vi "Configuration.vi"() -> ()   [LabVIEW 2018]
panel:
  out "error out":errorcluster
  in  "error in (no error)":errorcluster
  in  "Save":bool
  in  "Chromator COM":refnum<visa-resource-name>
  in  "Stop":bool
  in  "Merlin COM":refnum<visa-resource-name>
  in  "Source Meter COM":refnum<visa-resource-name>
  in  "Kaithely_PS COM":refnum<visa-resource-name>
  in  "Filter COM":refnum<visa-resource-name>
  # "Instrument Configuration"
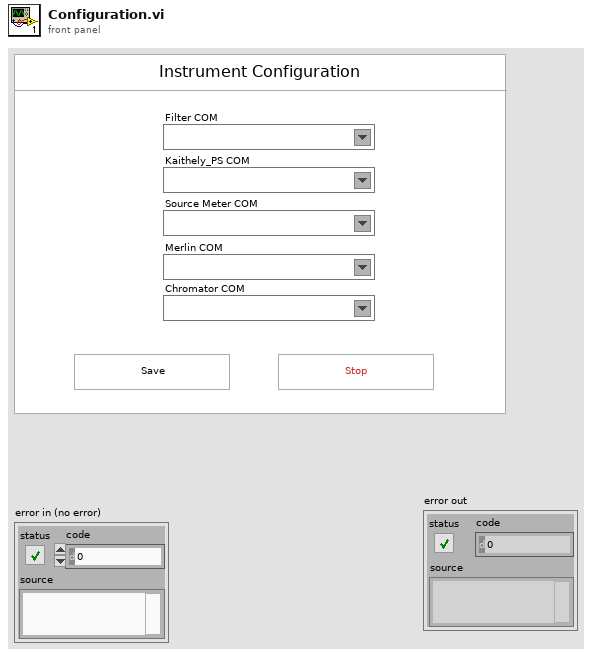
[diagram p1: front panel]
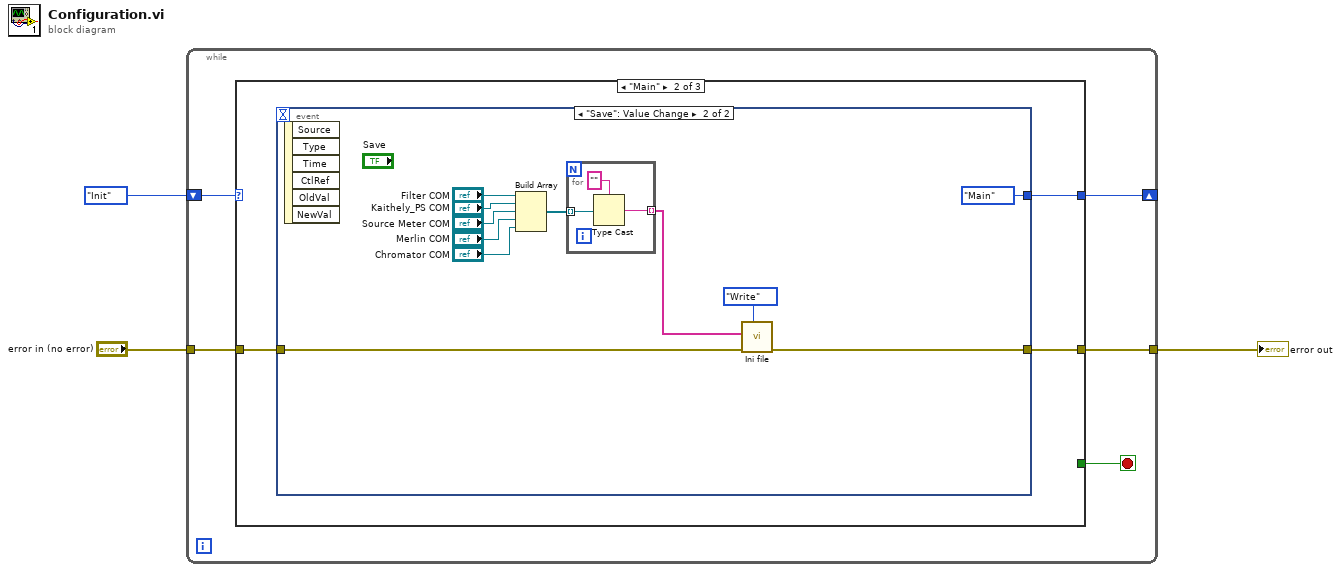
[diagram p0: block diagram]
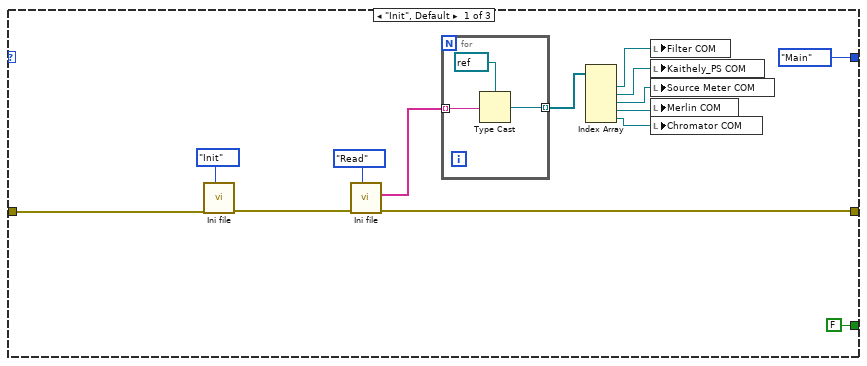
[diagram p2: hidden frame]
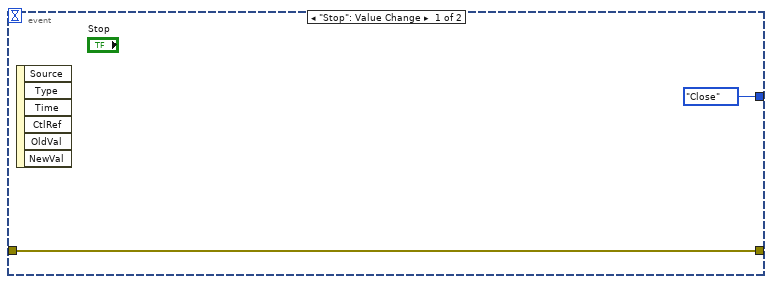
[diagram p3: hidden frame]
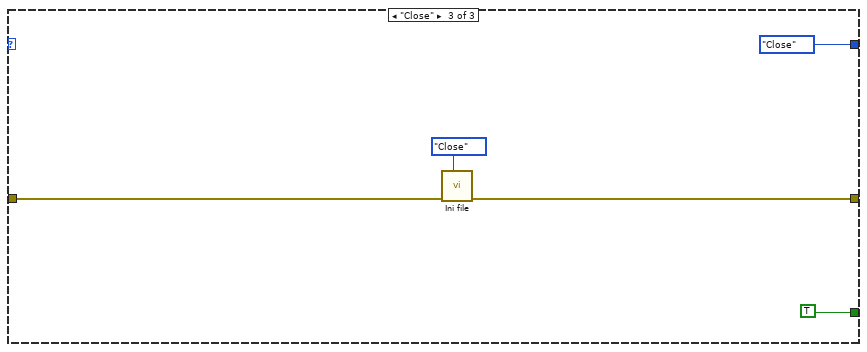
[diagram p4: hidden frame]
diagram:
  n1 = while {
    shift-right: [w7] -> _
    shift-left: enum16{"Init", "Main", "Close"}."Init" -> [w8]
    tunnel: "error in (no error)" -> [w5]
    tunnel: [w4] -> w1
    stop <- w6 stop-if-true
    n2 = case shown="\"Main\"" w8 {
      tunnel: [enum16{"Init", "Main", "Close"}."Main" w28 enum16{"Init", "Main", "Close"}."Close"] -> w7
      tunnel: [FALSE _ TRUE] -> w6
      tunnel: w5 -> [w20 w27 w47]
      tunnel: [w10 w26 w45] -> w4
      frame "Init", Default {
        n3 = call "Ini file.vi"("Command"=enum16{"Init", "Read", "Write", "Close"}."Init", "error in (no error)"=w20) -> ("error out"=w19:errorcluster)  [unwired: 8 in, 1 out]
        n4 = call "Ini file.vi"("Command"=enum16{"Init", "Read", "Write", "Close"}."Read", "error in (no error)"=w19) -> ("error out"=w10:errorcluster, "Data out"=w17:string[])  [unwired: 8 in]
        n5 = for {
          tunnel: w17 -> [w24] mode=indexing
          tunnel: [w23] -> w16 mode=indexing
          n6 = Type Cast(type=refnum<visa-resource-name> refnum ("VISA resource name"), x=w24) -> (*(type *) &x=w23:refnum<visa-resource-name>)
        }
        n7 = Index Array(array=w16) -> (element #1=w15:refnum<visa-resource-name>, element #2=w14:refnum<visa-resource-name>, element #3=w13:refnum<visa-resource-name>, element #4=w12:refnum<visa-resource-name>, element #5=w11:refnum<visa-resource-name>)  [unwired: 5 in]
        n8 = local write "Filter COM"(w15) -> ()
        n9 = local write "Kaithely_PS COM"(w14) -> ()
        n10 = local write "Source Meter COM"(w13) -> ()
        n11 = local write "Merlin COM"(w12) -> ()
        n12 = local write "Chromator COM"(w11) -> ()
      }
      frame "Main" {
        n13 = event shown="[1] \"Save\": Value Change" {
          selector: _ -> [_ _]
          dyn-events: _ -> [_ _]
          timeout: _ -> [_ _]
          tunnel: [enum16{"Init", "Main", "Close"}."Close" enum16{"Init", "Main", "Close"}."Main"] -> w28
          tunnel: w27 -> [w29 w33]
          tunnel: [w29 w32] -> w26
          event "Stop": Value Change {
            n14 = event-data() -> ()  [unwired: 1 in, 6 out]
          }
          event "Save": Value Change {
            n15 = event-data() -> ()  [unwired: 1 in, 6 out]
            n16 = Build Array("Filter COM", "Kaithely_PS COM", "Source Meter COM", "Merlin COM", "Chromator COM") -> (w36:refnum<visa-resource-name>[])
            n17 = for {
              tunnel: w36 -> [w44] mode=indexing
              tunnel: [w43] -> w31 mode=indexing
              n18 = Type Cast(type="", x=w44) -> (*(type *) &x=w43:string)
            }
            n19 = call "Ini file.vi"("Command"=enum16{"Init", "Read", "Write", "Close"}."Write", "error in (no error)"=w33, "Data in"=w31) -> ("error out"=w32:errorcluster)  [unwired: 7 in, 1 out]
          }
        }
      }
      frame "Close" {
        n20 = call "Ini file.vi"("Command"=enum16{"Init", "Read", "Write", "Close"}."Close", "error in (no error)"=w47) -> ("error out"=w45:errorcluster)  [unwired: 8 in, 1 out]
      }
    }
  }
  "error out" <- w1
